vi "SQL_Fetch All Data wo Ref.vi"(8 "error in (no error)":errorcluster, 10 "Table":string, 11 "SQL in":refnum<class "SQL.lvclass">) -> (0 "error out":errorcluster, 1 "columns":string[](array[string]), 2 "InitialData":string[][](array[string]), 3 "SQL out":refnum<class "SQL.lvclass">)   [LabVIEW 2012, in "SQL.lvclass"]
uses:
  SQL.lvclass
  <vilib>/addons/database/_DB Variant To Data/Database Variant To Data.xnode
  <vilib>/addons/database/NI_Database_API.lvlib
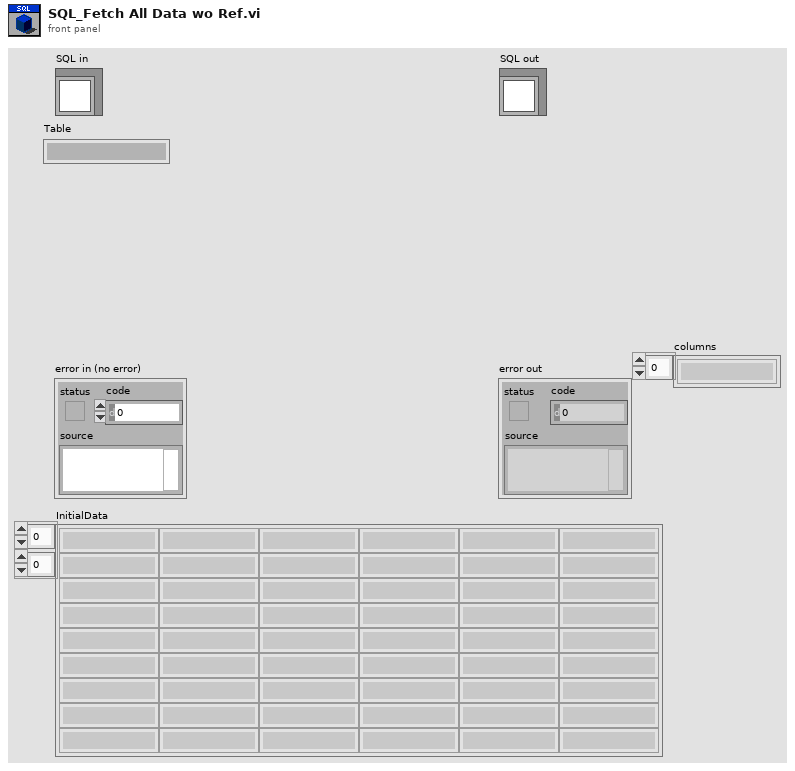
[diagram p1: front panel]
types:
  T1 = typedef "SQL.lvclass/ObjectAttributes.ctl" = cluster{"DB Connection Reference":T2}
  T2 = typedef "NI_Database_API.lvlib/Conn ObjectReference.ctl" = refnum<k1>
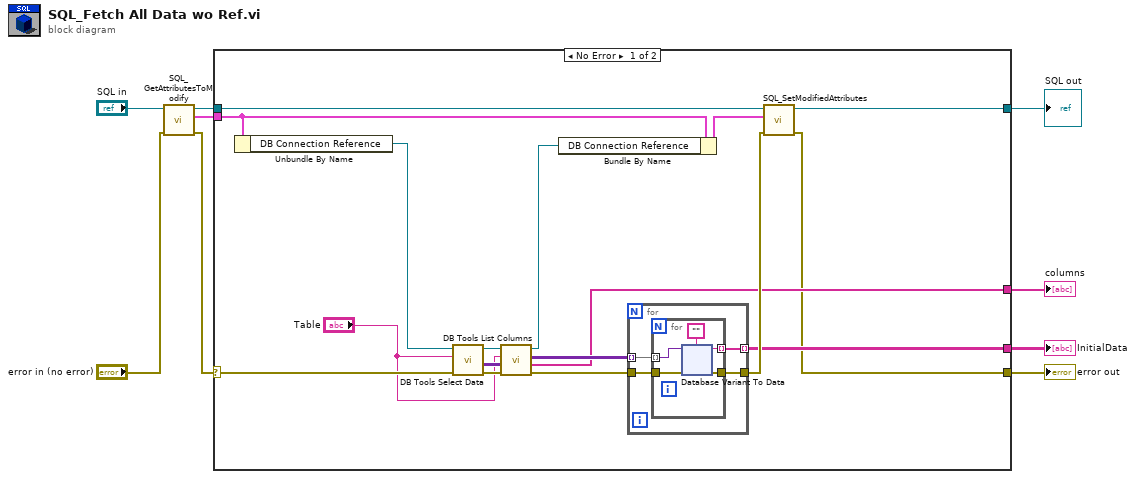
[diagram p0: block diagram]
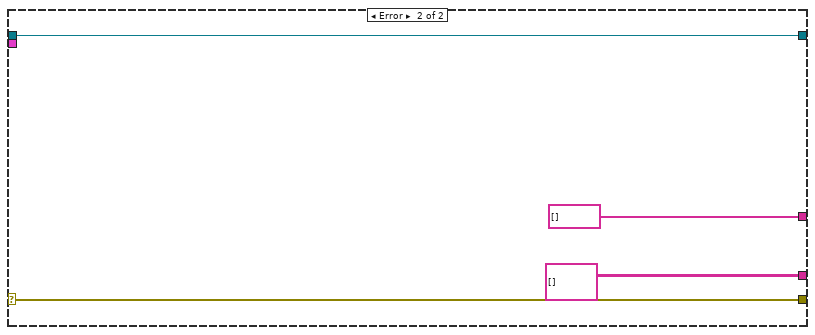
[diagram p2: hidden frame]
diagram:
  n1 = call "SQL_GetAttributesToModify.vi"("error in (no error)"="error in (no error)", "reference in"="SQL in") -> ("error out"=w2:errorcluster, "Attributes"=w5:T1, "reference out"=w6:refnum<class "SQL.lvclass">)  [unwired: 6 in, 1 out]
  n2 = case shown="No Error" w2 {
    selector: w2 -> [w22 w70]
    tunnel: [w10 w70] -> w9
    tunnel: [w24 w69] -> w8
    tunnel: w6 -> [w25 w69]
    tunnel: w5 -> [w21 _]
    tunnel: [w12 string[][] []] -> w4
    tunnel: [w11 string[] [] ("columns")] -> w1
    frame No Error {
      n3 = Unbundle By Name(w21) -> ("DB Connection Reference"=w19:T2)
      n4 = call <vilib>:"DB Tools Select Data.vi"("error in (no error)"=w22, "table"="Table", "connection reference"=w19) -> ("error out"=w17:errorcluster, "data"=w23:variant[][], "connection reference out"=w15:T2)  [unwired: 3 in]
      n5 = call <vilib>:"DB Tools List Columns.vi"("error in (no error)"=w17, "table"="Table", "connection reference"=w15) -> ("error out"=w16:errorcluster, "columns"=w11:string[], "connection reference out"=w13:T2)  [unwired: 1 in, 1 out]
      n6 = Bundle By Name(cluster=w21, "DB Connection Reference"=w13) -> (w20:T1)
      n7 = for {
        tunnel: w23 -> [w29] mode=indexing
        tunnel: [w28] -> w12 mode=indexing
        tunnel: [w27] -> w18
        tunnel: w16 -> [w26]
        n8 = for {
          tunnel: w29 -> [w33] mode=indexing
          tunnel: [w32] -> w28 mode=indexing
          tunnel: [w31] -> w27
          tunnel: w26 -> [w30]
          n9 = xnode "Database Variant To Data"("database variant"=w33, "error in"=w30, "type"="") -> ("data"=w32:string, "error out"=w31:errorcluster)
        }
      }
      n10 = call "SQL_SetModifiedAttributes.vi"("error in (no error)"=w18, "Attributes"=w20, "reference in"=w25) -> ("error out"=w10:errorcluster, "reference out"=w24:refnum<class "SQL.lvclass">)  [unwired: 7 in]
    }
    frame Error {
    }
  }
  "error out" <- w9
  "SQL out" <- w8
  "InitialData" <- w4
  "columns" <- w1
